vi "Const Configuration Default.vi"() -> (3 "Config":T1={"Language"={"Name"="English"}, "Path Config"={"Data Folder Path"=path "", "PNG Folder Path"=path ""}, "Image Viewer Config"={"Center Point"={"Size"=3, "Color"=16448250, "Show?"=TRUE}, "bp Point"={"Size"=3, "Color"=16711680, "Show?"=TRUE}, "w Point"={"Size"=3, "Color"=10546431, "Show?"=TRUE}, "b Box"={"Fill Color"=16752543, "Border Color"=16752543, "Show?"=TRUE}, "i Box"={"Fill Color"=16776305, "Border Color"=16776305, "Show?"=TRUE}, "o Point"={"Size"=3, "Color"=10546431, "Show?"=TRUE}, "c Point"={"Size"=3, "Color"=10546431, "Show?"=TRUE}}})   [LabVIEW 2018, in "Main Panel.lvlib" / "Main Panel.lvclass"]
uses:
  Main Panel.lvclass
  Const Configuration.ctl
  Const Path Setting.ctl
  Const Image Viewer Setting.ctl
  Framework/Framework/Framework.lvclass
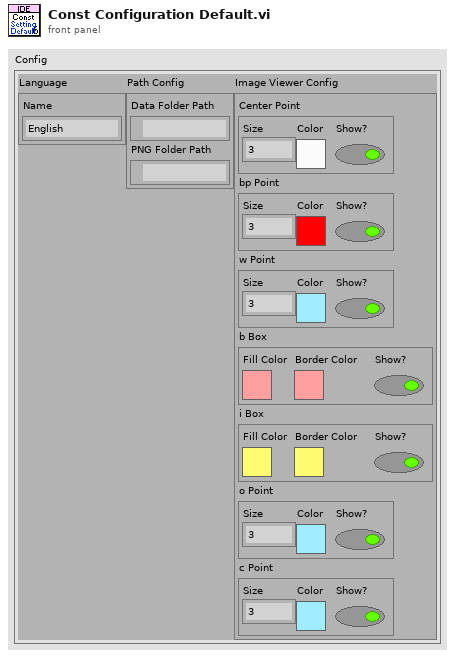
[diagram p1: front panel]
types:
  T1 = typedef "Main Panel.lvlib/Main Panel.lvclass/Const Configuration.ctl" = cluster{"Language":cluster{"Name":string}, "Path Config":T2, "Image Viewer Config":T3}
  T2 = typedef "Main Panel.lvlib/Main Panel.lvclass/Const Path Setting.ctl" = cluster{"Data Folder Path":path, "PNG Folder Path":path}
  T3 = typedef "Main Panel.lvlib/Main Panel.lvclass/Const Image Viewer Setting.ctl" = cluster{"Center Point":cluster{"Size":i32, "Color":u32, "Show?":bool}, "bp Point":cluster{"Size":i32, "Color":u32, "Show?":bool}, "w Point":cluster{"Size":i32, "Color":u32, "Show?":bool}, "b Box":cluster{"Fill Color":u32, "Border Color":u32, "Show?":bool}, "i Box":cluster{"Fill Color":u32, "Border Color":u32, "Show?":bool}, "o Point":cluster{"Size":i32, "Color":u32, "Show?":bool}, "c Point":cluster{"Size":i32, "Color":u32, "Show?":bool}}
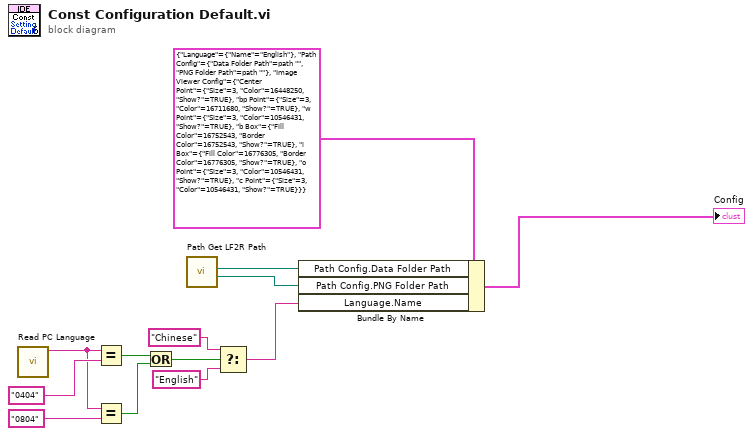
[diagram p0: block diagram]
diagram:
  n1 = call "Read PC Language.vi"() -> ("Language Hex Code"=w8:string)  [unwired: 11 in]
  n2 = Equal?(x=w8, y="0404") -> (x = y?=w6:bool)
  n3 = Equal?(x=w8, y="0804") -> (x = y?=w5:bool)
  n4 = Or(x=w6, y=w5) -> (x .or. y?=w4:bool)
  n5 = call "Path Get LF2R Path.vi"() -> ("PNG Path"=w11:path, "Data Path"=w12:path)  [unwired: 7 in, 3 out]
  n6 = Select(t="Chinese" ("y"), s=w4, f="English" ("y")) -> (s? t:f=w1:string)
  n7 = Bundle By Name(cluster=T1 {"Language"={"Name"="English"}, "Path Config"={"Data Folder Path"=path "", "PNG Folder Path"=path ""}, "Image Viewer Config"={"Center Point"={"Size"=3, "Color"=16448250, "Show?"=TRUE}, "bp Point"={"Size"=3, "Color"=16711680, "Show?"=TRUE}, "w Point"={"Size"=3, "Color"=10546431, "Show?"=TRUE}, "b Box"={"Fill Color"=16752543, "Border Color"=16752543, "Show?"=TRUE}, "i Box"={"Fill Color"=16776305, "Border Color"=16776305, "Show?"=TRUE}, "o Point"={"Size"=3, "Color"=10546431, "Show?"=TRUE}, "c Point"={"Size"=3, "Color"=10546431, "Show?"=TRUE}}} ("Config 2"), "Path Config.Data Folder Path"=w12, "Path Config.PNG Folder Path"=w11, "Language.Name"=w1) -> (→"Config":T1)
